vi "number1_sub1-configure data acquisition.vi"(5 "OK Button":bool) -> ()   [LabVIEW 2014]
uses:
  number1_global.vi
panel:
  in  "samples per acquisition":dbl=10000.0
  in  "sampling rate (samples/sec)":dbl=1000.0
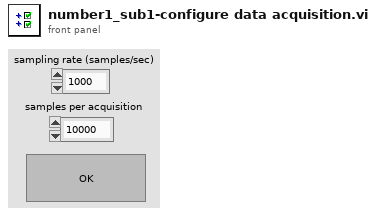
[diagram p1: front panel]
types:
  T1 = enum32{"Invalid", "Standard", "Closed", "Hidden", "Minimized", "Maximized"}
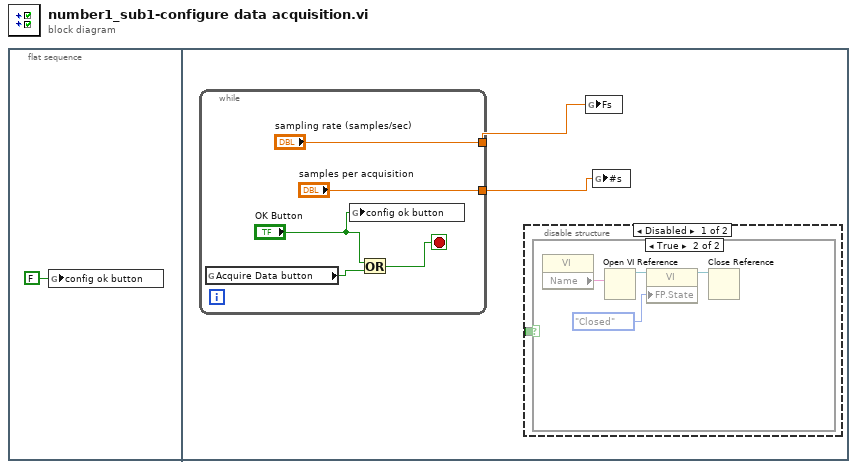
[diagram p0: block diagram]
diagram:
  n1 = flat-sequence {
    frame #0 {
      n2 = global write "number1_global.vi" "config ok button"(FALSE ("config ok button")) -> ()
    }
    frame #1 {
      n3 = while {
        tunnel: ["sampling rate (samples/sec)"] -> w3
        tunnel: ["samples per acquisition"] -> w2
        stop <- w9 stop-if-true
        n4 = global read "number1_global.vi" "Acquire Data button"() -> (w11:bool)
        n5 = global write "number1_global.vi" "config ok button"("OK Button") -> ()
        n6 = Or(x="OK Button", y=w11) -> (x .or. y?=w9:bool)
      }
      n7 = disable-structure shown="Disabled" {
        disable-tunnel: _ -> [w4 _]
        frame Disabled {
          n8 = case shown="True" w4 {
            frame False {
            }
            frame True {
              n9 = property class="VI"() -> ("Name"=w8:string)  [unwired: 2 in, 2 out]
              n10 = Open VI Reference(vi path=w8) -> (vi reference=w7:refnum<vi>)  [unwired: 5 in, 1 out]
              n11 = property class="VI"(reference=w7, "FP.State"=T1."Closed" ("Front Panel Window:State")) -> (reference out=w6:refnum<vi>)  [unwired: 1 in, 1 out]
              n12 = Close Reference(reference=w6) -> ()  [unwired: 1 in, 1 out]
            }
          }
        }
        frame Enabled {
        }
      }
      n13 = global write "number1_global.vi" "Fs"(w3) -> ()
      n14 = global write "number1_global.vi" "#s"(w2) -> ()
    }
  }
